vi "Plot_Current_Measurement_Data.vi"() -> ()   [LabVIEW 2015]
uses:
  Anemometry Sub Vis/Globals/Meas_global.vi
panel:
  in  "Index 2 scale":dbl=1.0
  in  "Index 2":i32
  in  "Index1":i32
  out "XY Graph":cluster{"Time (s)":dbl[], "Eng Values":dbl[]}[](graph)
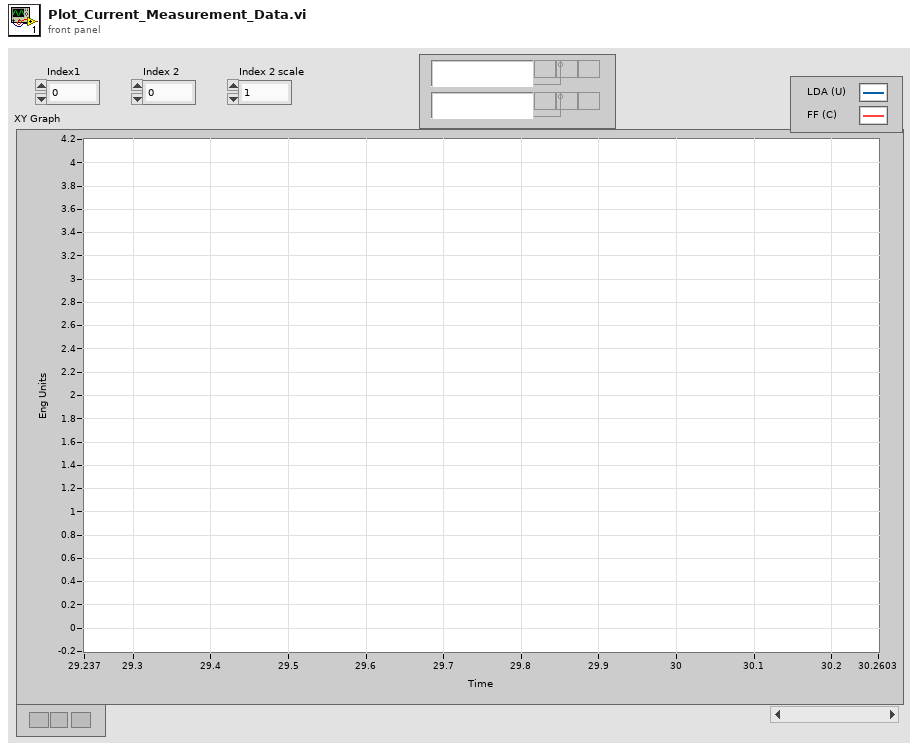
[diagram p1: front panel]
types:
  T1 = typedef "Time_Trace_Cluster.ctl" = cluster{"Weighting":dbl[], "Time (s)":dbl[], "Voltage":dbl[], "Eng Values":dbl[]}
  T2 = typedef "Analysis_info_cluster.ctl" = cluster{"Colour":u32, "Inst type":T3, "Inst name":string, "Symbol":string, "Code name":string, "Extra Info":string, "Inst Array":T4, "Extra Titles":string[], "Extra Values":string[], "U":dbl, "u^2":dbl, "u^3":dbl, "u^4":dbl, "Skew_u":dbl, "Kurt_u":dbl, "Sd Error in Mean":dbl, "% u'/U":dbl, "X":dbl, "Y":dbl, "Z":dbl, "Timescale integral to 25%":dbl, "Sd Error in Variance":dbl, "Calib File":path, "Calib Constants":dbl[], "Output Position":bool, "Full Stats":bool, "Av Sampling Rate":dbl, "Av No of Samples":dbl, "Total Meas Time (s)":dbl, "ADAM Ch Name":string}
  T3 = typedef "Inst_type.ctl" = enum16{"Propeller anemometer", "Raw voltage", "Pressure Transducer", "Pitot-static tube", "Preston tube", "Hot wire", "Cross wire 1", "Cross wire 2", "Generic Linear", "Generic Polynomial", "Generic BackPoly", "Fast FID", "Thermocouple", "Cold wire", "Pulsed Wire", "LDA Vel", "LDA Tran time", "LDA Arr time", "Microphone"}
  T4 = typedef "Instrument_Array.ctl" = enum16{"PWA", "LDA", "Analogue"}
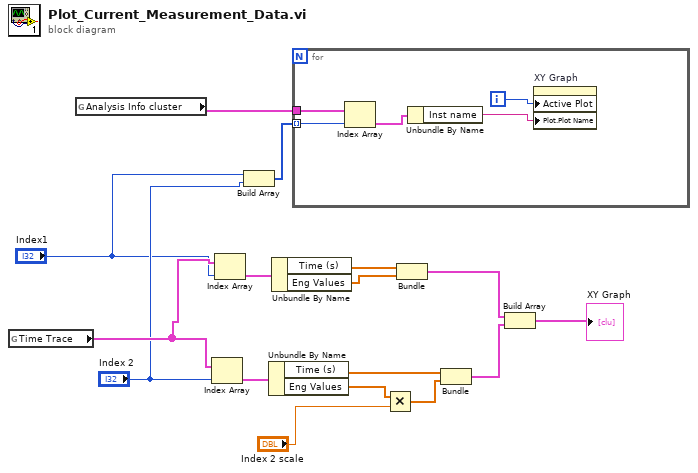
[diagram p0: block diagram]
diagram:
  n1 = global read "Meas_global.vi" "Time Trace"() -> (w11:T1[])
  n2 = global read "Meas_global.vi" "Analysis Info cluster"() -> (w1:T2[])
  n3 = Index Array(array=w11, index="Index 2") -> (element=w16:T1)
  n4 = Index Array(array=w11, index="Index1") -> (element=w12:T1)
  n5 = Build Array("Index1", "Index 2") -> (w2:i32[])
  n6 = Unbundle By Name(w16) -> ("Time (s)"=w15:dbl[], "Eng Values"=w10:dbl[])
  n7 = Unbundle By Name(w12) -> ("Time (s)"=w13:dbl[], "Eng Values"=w14:dbl[])
  n8 = for {
    tunnel: w2 -> [w20] mode=indexing
    tunnel: w1 -> [w19]
    i -> [w17]
    n9 = Index Array(array=w19, index=w20) -> (element=w18:T2)
    n10 = Unbundle By Name(w18) -> ("Inst name"=w21:string)
    n11 = property on="XY Graph" class="XYGraph (strict)"("Active Plot"=w17, "Plot.Plot Name"=w21) -> ()  [unwired: 2 in, 2 out]
  }
  n12 = Multiply(x=w10, y="Index 2 scale") -> (x*y=w8:dbl[])
  n13 = Bundle("Time (s)"=w13, "Eng Values"=w14) -> (w6:cluster{"Time (s)":dbl[], "Eng Values":dbl[]})  [unwired: 1 in]
  n14 = Bundle("Time (s)"=w15, w8) -> (w7:cluster{"Time (s)":dbl[], dbl[]})  [unwired: 1 in]
  n15 = Build Array(w6, w7) -> (→"XY Graph":cluster{"Time (s)":dbl[], "Eng Values":dbl[]}[])
